vi "autonSample.vi"(0 "Auton Array":dbl[][](array[numeric]), 5 "MeasuredHeading":dbl, 9 "EncoderDistance":dbl) -> (4 "Left Drive":dbl(knob) scale=-1.0..1.0, 6 "Right Drive":dbl(knob) scale=-1.0..1.0, 8 "Ramp ACT motor":dbl, 10 "Turret Rotation":dbl, 14 "Harvester":dbl, 15 "Shooter motor output":dbl)   [LabVIEW 2011]
uses:
  Robot Global Data.vi
  <vilib>/addons/control/pid/pid.llb/PID (DBL).vi
  <vilib>/addons/control/pid/NI_PID_pid.lvlib
panel:
  out "Numeric":i16
  out "Tzero":i64
  out "AccumDist":dbl
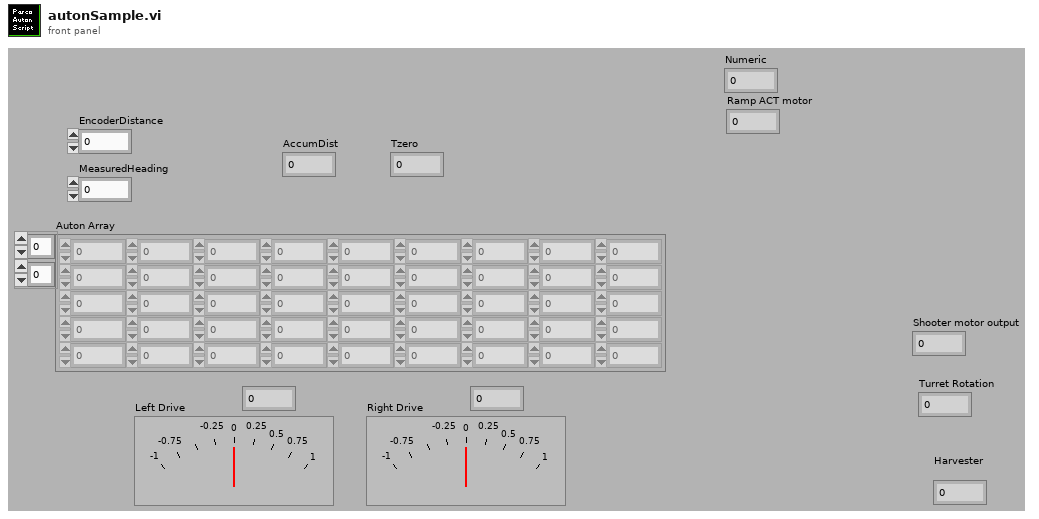
[diagram p1: front panel]
types:
  T1 = cluster{"proportional gain (Kc)":dbl, "integral time (Ti, min)":dbl, "derivative time (Td, min)":dbl}
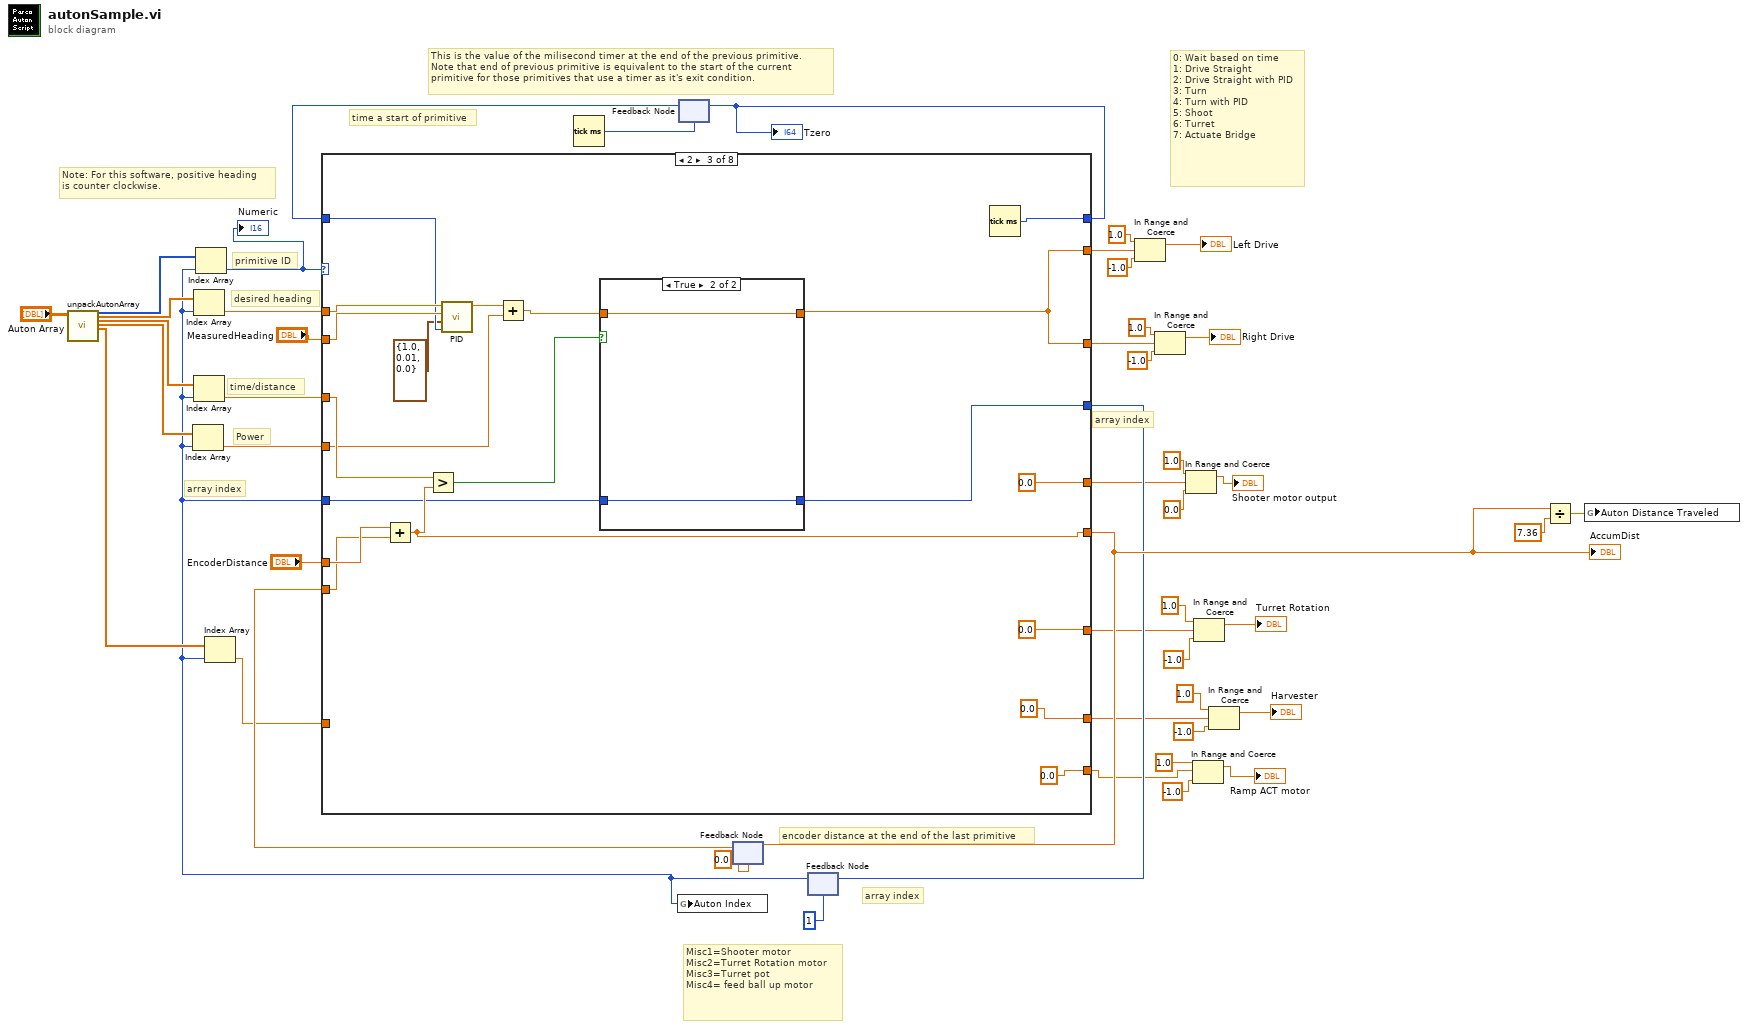
[diagram p0: block diagram]
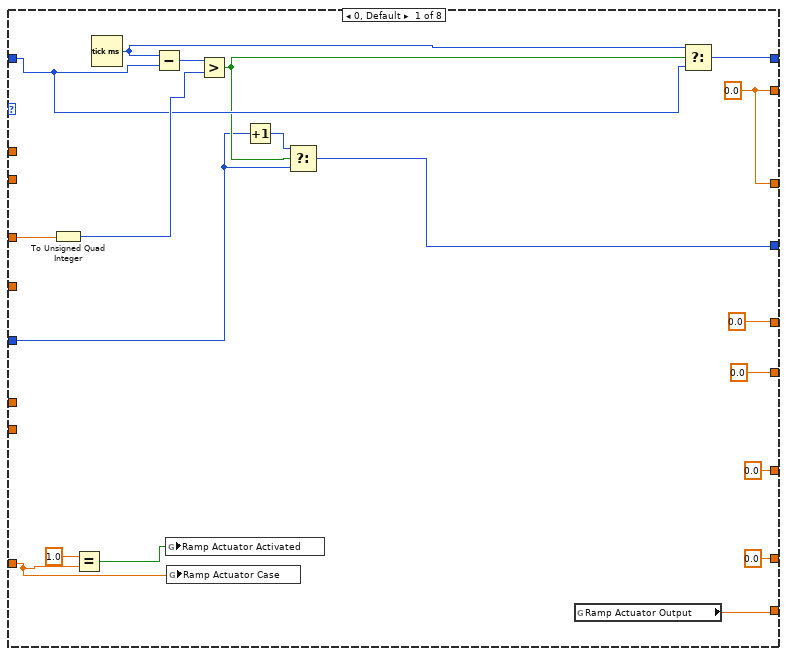
[diagram p2: hidden frame]
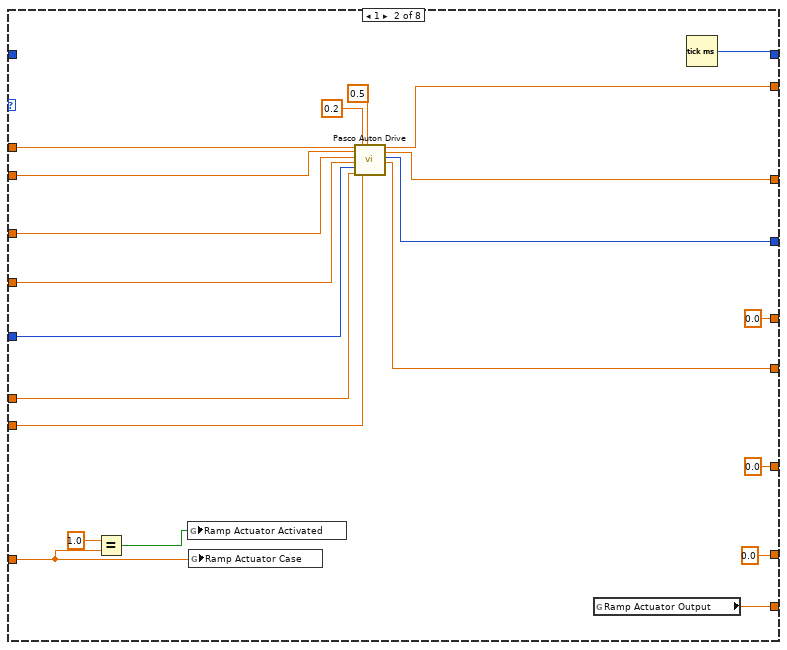
[diagram p3: hidden frame]
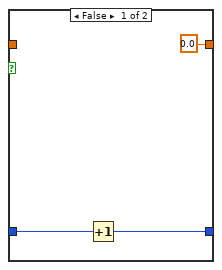
[diagram p4: hidden frame]
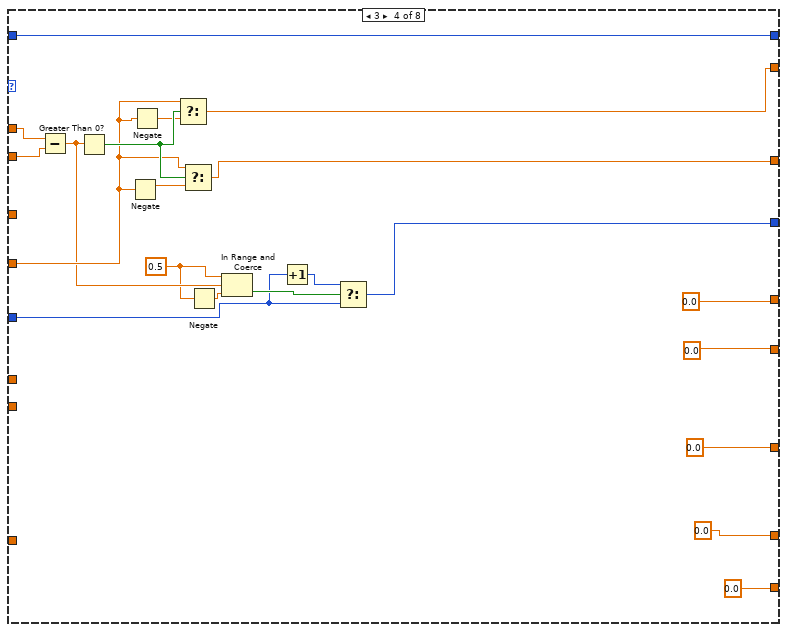
[diagram p5: hidden frame]
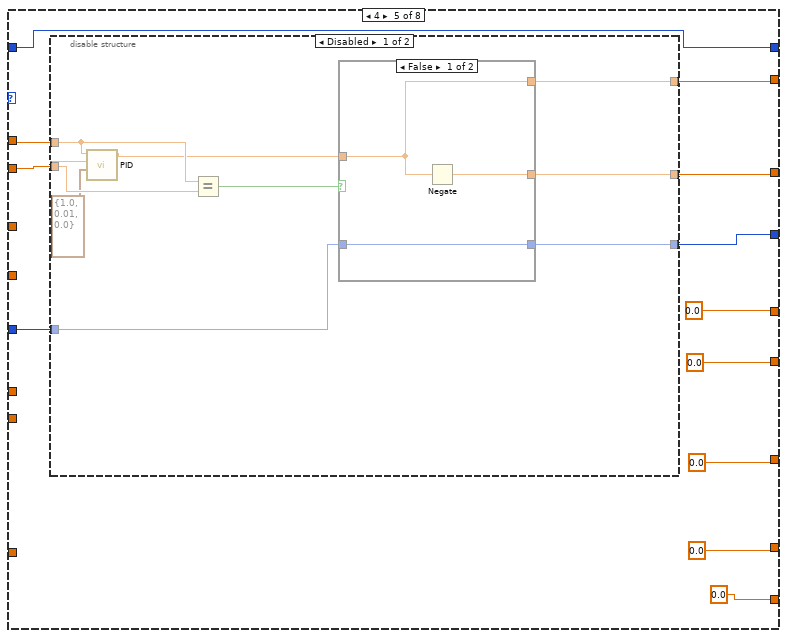
[diagram p6: hidden frame]
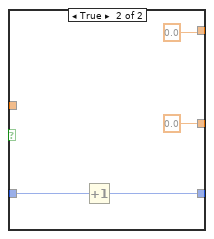
[diagram p7: hidden frame]
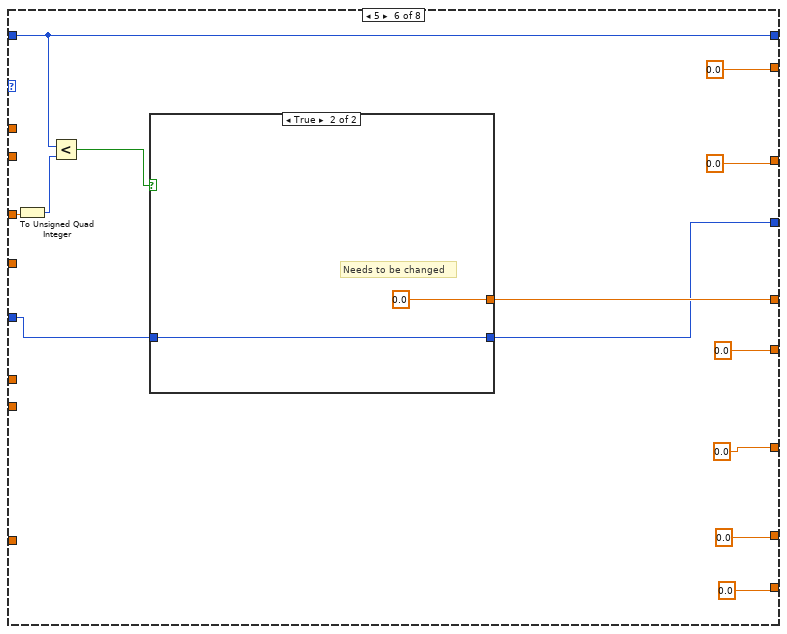
[diagram p9: hidden frame]
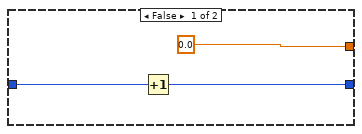
[diagram p10: hidden frame]
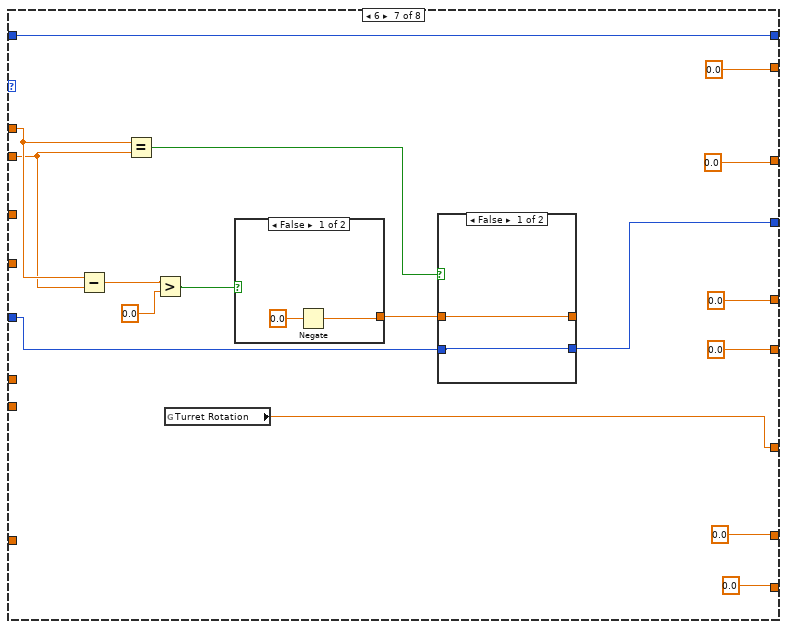
[diagram p11: hidden frame]
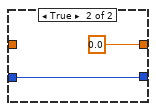
[diagram p12: hidden frame]
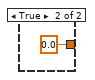
[diagram p13: hidden frame]
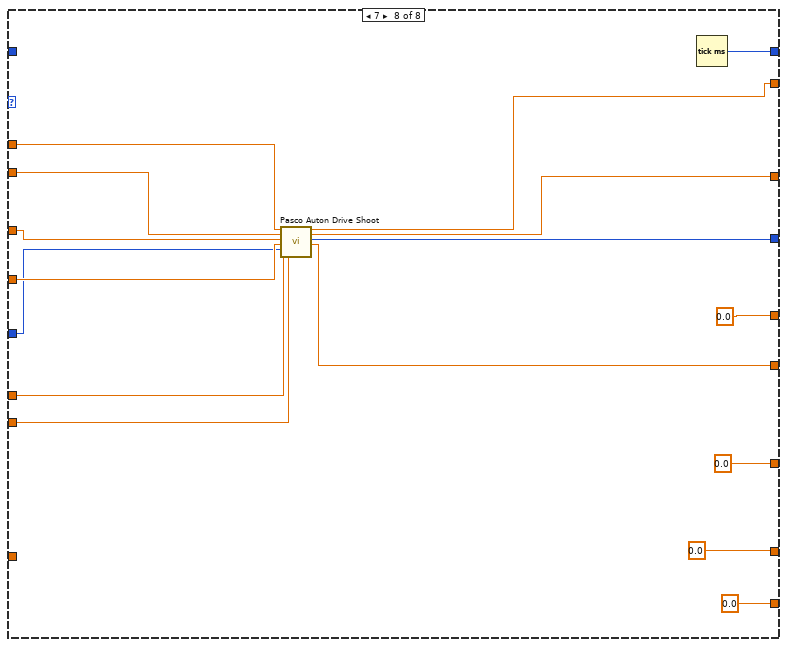
[diagram p14: hidden frame]
diagram:
  # "Misc1=Shooter motor\nMisc2=Turret Rotation motor\nMisc3=Turret pot\nMisc4= feed ball up motor"
  # "0: Wait based on time\n1: Drive Straight\n2: Drive Straight with PID\n3: Turn\n4: Turn with PID\n5: Shoot\n6: Turret\n7: Actuate Bridge"
  # "encoder distance at the end of the last primitive"
  # "Note: For this software, positive heading\nis counter clockwise."
  # "time a start of primitive"
  # "array index"
  # "array index"
  # "This is the value of the milisecond timer at the end of the previous primitive.\nNote that end of previous primitive is equivalent to the start of the current\nprimitive for those primitives that use a timer as it's exit condition."
  # "Power"
  # "array index"
  # "desired heading"
  # "primitive ID"
  # "time/distance"
  n1 = call "unpackAutonArray.vi"("all rows"="Auton Array") -> ("Primitive"=w47:i16[], "Left Drive"=w30:dbl[], "Right Drive"=w31:dbl[], "Ramp ACT"=w28:dbl[], "Conveyor"=w7:dbl[])  [unwired: 1 in, 21 out]
  n2 = Tick Count (ms)() -> (millisecond timer value=w42:u32)
  n3 = feedback #1(w42) -> (w46:u32)
  n4 = feedback #2(0.0 ("EncoderDistance")) -> (w27:dbl)
  n5 = feedback #3(1) -> (w6:i32)
  n6 = Index Array(array=w28, index=w6) -> (element=w44:dbl)
  n7 = Index Array(array=w30, index=w6) -> (element=w29:dbl)
  n8 = Index Array(array=w31, index=w6) -> (element=w45:dbl)
  n9 = Index Array(array=w47, index=w6) -> (element=w8:i16)
  "Numeric" <- w8
  n10 = Index Array(array=w7, index=w6) -> (element=w5:dbl)
  n11 = case shown="2" w8 {
    tunnel: [w55 w69 w101 w116 w140 w170 w193 w206] -> w22
    tunnel: w6 -> [w56 w74 w102 w118 w139 w171 w194 w212]
    tunnel: [w67 w87 w108 w114 w146 w165 w192 w218] -> w32
    tunnel: w46 -> [w63 _ w95 w114 w146 w165 w192 _]
    tunnel: w45 -> [w65 w76 w104 _ _ w175 _ w214]
    tunnel: w29 -> [_ w78 w96 w130 w136 _ w197 w216]
    tunnel: [w54 w71 w103 w124 w141 0.0 0.0 w209] -> w40
    tunnel: [w54 w70 w103 w123 w142 0.0 0.0 w208] -> w33
    tunnel: w44 -> [_ w75 w92 w126 _ _ _ w213]
    tunnel: "EncoderDistance" -> [_ w73 w107 _ _ _ _ w210]
    tunnel: "MeasuredHeading" -> [_ w77 w97 w129 w137 _ w183 w215]
    tunnel: [0.0 ("Encoder total") w68 w105 0.0 0.0 0.0 0.0 w207] -> w24
    tunnel: w27 -> [_ w72 w106 _ _ _ _ w211]
    tunnel: [0.0 ("Misc1  OUT") 0.0 ("Misc1  OUT") 0.0 0.0 0.0 w172 0.0 0.0 ("Misc1  OUT")] -> w18
    tunnel: [0.0 ("Misc2 OUT") 0.0 ("Misc2 OUT") 0.0 0.0 0.0 0.0 w182 0.0 ("Misc1  OUT")] -> w14
    tunnel: [0.0 ("Misc4 OUT") 0.0 0.0 0.0 0.0 0.0 0.0 0.0] -> w10
    tunnel: w5 -> [w50 w84 _ _ _ _ _ _]
    tunnel: [w49 w81 0.0 ("Ramp Actuator Output") 0.0 ("Ramp Actuator Output") 0.0 ("Ramp Actuator Output") 0.0 ("Ramp Actuator Output") 0.0 ("Ramp Actuator Output") 0.0 ("Ramp Actuator Output")] -> w4
    frame 0, Default {
      w54 = 0.0 ("Numeric")
      n12 = To Unsigned Quad Integer(1:w65) -> (0:w64:u64)
      n13 = Equal?(x=1.0, y=w50) -> (x = y?=w51:bool)
      n14 = Tick Count (ms)() -> (millisecond timer value=w62:u32)
      n15 = Subtract(x=w62, y=w63) -> (x-y=w66:u32)
      n16 = global write "Robot Global Data.vi" "Ramp Actuator Activated"(w51) -> ()
      n17 = global write "Robot Global Data.vi" "Ramp Actuator Case"(w50) -> ()
      n18 = Greater?(x=w66, y=w64) -> (0:w58:bool)
      n19 = Increment(x=w56) -> (x+1=w57:i32)
      n20 = Select(t=w57, s=w58, f=w56) -> (s? t:f=w55:i32)
      n21 = global read "Robot Global Data.vi" "Ramp Actuator Output"() -> (w49:dbl)
      n22 = Select(t=w62, s=w58, f=w63) -> (s? t:f=w67:u32)
    }
    frame 1 {
      n23 = Equal?(x=1.0, y=w84) -> (x = y?=w82:bool)
      n24 = global write "Robot Global Data.vi" "Ramp Actuator Activated"(w82) -> ()
      n25 = global write "Robot Global Data.vi" "Ramp Actuator Case"(w84) -> ()
      n26 = call "Pasco Auton Drive.vi"("Desired Heading"=w78, "Measured Heading"=w77, "Time/Distance"=w76, "Power"=w75, "Array Index"=w74, "Encoder Distance"=w73, "Increase Power To Each Side"=0.2, "Returned Encoder Distance"=w72, "Alloted Off Amount"=0.5) -> ("Left Drive"=w71:dbl, "Right Drive"=w70:dbl, "Array Index"=w69:i32, "Encoder Out"=w68:dbl)  [unwired: 7 in]
      n27 = global read "Robot Global Data.vi" "Ramp Actuator Output"() -> (w81:dbl)
      n28 = Tick Count (ms)() -> (millisecond timer value=w87:u32)
    }
    frame 2 {
      n29 = Add(x=w107, y=w106) -> (x+y=w105:dbl)
      n30 = Greater?(x=w104, y=w105) -> (0:w94:bool)
      n31 = call-poly <vilib>:"PID.vi"("dt (s)"=w95, "PID gains"=T1 {"proportional gain (Kc)"=1.0, "integral time (Ti, min)"=0.01, "derivative time (Td, min)"=0.0}, "process variable"=w97, "setpoint"=w96) -> ("output"=w91:dbl)  [unwired: 6 in, 1 out]
      n32 = Add(x=w91, y=w92) -> (x+y=w90:dbl)
      n33 = case shown="True" w94 {
        tunnel: [0.0 w113] -> w103
        tunnel: w90 -> [_ w113]
        tunnel: w102 -> [w111 w112]
        tunnel: [w110 w112] -> w101
        frame False {
          n34 = Increment(x=w111) -> (x+1=w110:i32)
        }
        frame True {
        }
      }
      n35 = Tick Count (ms)() -> (millisecond timer value=w108:u32)
    }
    frame 3 {
      w121 = 0.5 ("upper limit")
      n36 = Subtract(x=w130, y=w129) -> (x-y=w122:dbl)
      n37 = Greater Than 0?(x=w122) -> (x > 0?=w128:bool)
      n38 = Negate(x=w126) -> (-x=w127:dbl)
      n39 = Negate(x=w126) -> (-x=w125:dbl)
      n40 = Select(t=w126, s=w128, f=w125) -> (s? t:f=w124:dbl)
      n41 = Select(t=w126, s=w128, f=w127) -> (s? t:f=w123:dbl)
      n42 = Negate(x=w121) -> (-x=w120:dbl)
      n43 = In Range and Coerce(upper limit=w121, x=w122, lower limit=w120) -> (In Range?=w119:bool)  [unwired: 1 out]
      n44 = Increment(x=w118) -> (x+1=w117:i32)
      n45 = Select(t=w117, s=w119, f=w118) -> (s? t:f=w116:i32)
    }
    frame 4 {
      n46 = disable-structure shown="Disabled" {
        disable-tunnel: [w155 _] -> w142
        disable-tunnel: [w154 _] -> w141
        disable-tunnel: [w153 _] -> w140
        disable-tunnel: w139 -> [w152 _]
        disable-tunnel: w137 -> [w150 _]
        disable-tunnel: w136 -> [w149 _]
        frame Disabled {
          n47 = call-poly <vilib>:"PID.vi"("PID gains"=T1 {"proportional gain (Kc)"=1.0, "integral time (Ti, min)"=0.01, "derivative time (Td, min)"=0.0}, "process variable"=w150, "setpoint"=w149) -> ("output"=w148:dbl)  [unwired: 7 in, 1 out]
          n48 = Equal?(x=w149, y=w150) -> (x = y?=w151:bool)
          n49 = case shown="False" w151 {
            tunnel: w148 -> [w157 _]
            tunnel: [w158 0.0] -> w155
            tunnel: [w157 0.0] -> w154
            tunnel: [w156 w161] -> w153
            tunnel: w152 -> [w156 w162]
            frame False {
              n50 = Negate(x=w157) -> (-x=w158:dbl)
            }
            frame True {
              n51 = Increment(x=w162) -> (x+1=w161:i32)
            }
          }
        }
        frame Enabled {
        }
      }
    }
    frame 5 {
      n52 = To Unsigned Quad Integer(1:w175) -> (0:w173:u64)
      n53 = Less?(x=w165, y=w173) -> (x < y?=w174:bool)
      n54 = case shown="True" w174 {
        tunnel: [0.0 0.0] -> w172
        tunnel: w171 -> [w177 w180]
        tunnel: [w176 w180] -> w170
        frame False {
          n55 = Increment(x=w177) -> (x+1=w176:i32)
        }
        frame True {
          # "Needs to be changed"
        }
      }
    }
    frame 6 {
      n56 = Subtract(x=w197, y=w183) -> (x-y=w185:dbl)
      n57 = Equal?(x=w197, y=w183) -> (x = y?=w196:bool)
      n58 = Greater?(x=w185, y=0.0) -> (0:w186:bool)
      n59 = global read "Robot Global Data.vi" "Turret Rotation"() -> (w182:dbl)
      n60 = case shown="False" w186 {
        tunnel: [w203 0.0] -> w195
        frame False {
          n61 = Negate(x=0.0) -> (-x=w203:dbl)
        }
        frame True {
        }
      }
      n62 = case shown="False" w196 {
        tunnel: [w199 0.0] -> _
        tunnel: w195 -> [w199 _]
        tunnel: w194 -> [w198 w201]
        tunnel: [w198 w201] -> w193
        frame False {
        }
        frame True {
        }
      }
    }
    frame 7 {
      n63 = call "Pasco Auton Drive Shoot.vi"("Desired Heading"=w216, "Actual Heading"=w215, "time/distance"=w214, "Power"=w213, "Array"=w212, "Encoder total"=w210, "Encoder Return"=w211) -> ("Left Drive"=w209:dbl, "Right Drive"=w208:dbl, "Array Out"=w206:i32, "Encoder total"=w207:dbl)  [unwired: 9 in]
      n64 = Tick Count (ms)() -> (millisecond timer value=w218:u32)
    }
  }
  "AccumDist" <- w24
  "Tzero" <- w32
  n65 = global write "Robot Global Data.vi" "Auton Index"(w6) -> ()
  n66 = feedback-in #1(w32) -> ()
  n67 = feedback-in #2(w24) -> ()
  n68 = feedback-in #3(w22) -> ()
  n69 = In Range and Coerce(upper limit=1.0, x=w40, lower limit=-1.0) -> (coerced(x)=→"Left Drive":dbl)  [unwired: 1 out]
  n70 = In Range and Coerce(upper limit=1.0, x=w33, lower limit=-1.0) -> (coerced(x)=→"Right Drive":dbl)  [unwired: 1 out]
  n71 = In Range and Coerce(upper limit=1.0, x=w18, lower limit=0.0) -> (coerced(x)=→"Shooter motor output":dbl)  [unwired: 1 out]
  n72 = In Range and Coerce(upper limit=1.0, x=w4, lower limit=-1.0) -> (coerced(x)=→"Ramp ACT motor":dbl)  [unwired: 1 out]
  n73 = In Range and Coerce(upper limit=1.0, x=w14, lower limit=-1.0) -> (coerced(x)=→"Turret Rotation":dbl)  [unwired: 1 out]
  n74 = In Range and Coerce(upper limit=1.0, x=w10, lower limit=-1.0) -> (coerced(x)=→"Harvester":dbl)  [unwired: 1 out]
  n75 = Divide(x=w24, y=7.36) -> (x/y=w9:dbl)
  n76 = global write "Robot Global Data.vi" "Auton Distance Traveled"(w9) -> ()
